vi "Get Sensor Calibration Coeffs.vi"(11 "Select Probe":i32) -> (2 "CalibrCoefArray":dbl[](array[numeric]), 3 "Total Pixels":u16)   [LabVIEW 2015, in "Tool Cfg.lvlib"]
uses:
  Tool Cfg.lvlib
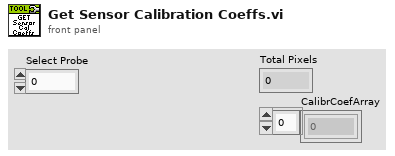
[diagram p1: front panel]
types:
  T1 = typedef "Tool Cfg.lvlib/_SensorConfigParams Cluster--typedef.ctl" = cluster{"Total Pixels":u16, "Positive  Peaks":bool, "CalibrCoefArray":dbl[], "Start Idx":u16, "End Idx":u16}
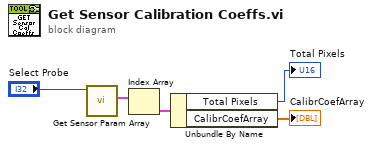
[diagram p0: block diagram]
diagram:
  n1 = call "Get Sensor Param Array.vi"("Select Probe"="Select Probe") -> ("Sensor Block.SensorCfgParams Array"=w4:T1[])  [unwired: 9 in, 1 out]
  n2 = Index Array(array=w4) -> (element=w3:T1)  [unwired: 1 in]
  n3 = Unbundle By Name(w3) -> ("Total Pixels"=→"Total Pixels":u16, "CalibrCoefArray"=→"CalibrCoefArray":dbl[])
